vi "ReplaceStringLUT.vi"(9 "Replacement":string[](array[string])=["0.5", "0.5", "Inf"], 10 "Search List":string[](array[string])=["1/2", "½", "∞"], 11 "String In":string) -> (3 "String Out":string)   [LabVIEW 2023]
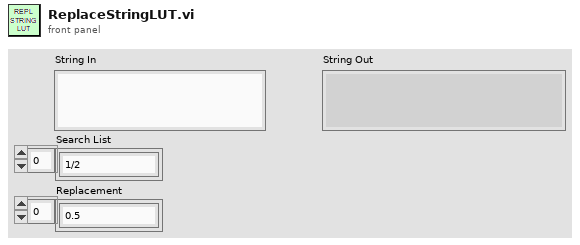
[diagram p1: front panel]
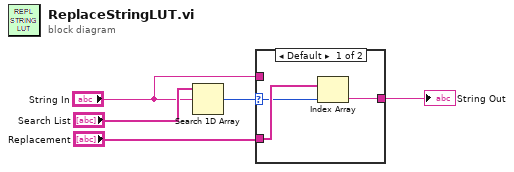
[diagram p0: block diagram]
diagram:
  n1 = Search 1D Array(1D array="Search List", element="String In") -> (index of element=w4:i32)  [unwired: 1 in]
  n2 = case shown="Default" w4 {
    selector: w4 -> [w7 _]
    tunnel: "Replacement" -> [w8 _]
    tunnel: [w6 w9] -> w1
    tunnel: "String In" -> [_ w9]
    frame Default {
      n3 = Index Array(array=w8, index=w7) -> (element=w6:string)
    }
    frame -1 {
    }
  }
  "String Out" <- w1
